vi "Resolve Link.vi"   [LabVIEW 2021, in "Field_RnD_Services_LIBSSH2_Toolkit.lvlib" / "SFTP.lvclass"]
doc: "Gets the absolute path of a symbolic or real link's target, a.k.a. source."
uses:
  SFTP.lvclass
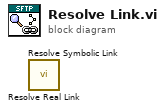
[diagram p0: block diagram]
diagram:
  n1 = call "Resolve Real Link.vi"() -> ()  [unwired: 9 in, 3 out]
  n2 = call "Resolve Symbolic Link.vi"() -> ()  [unwired: 9 in, 3 out]
